vi "Execute Menu Item.vi"(7 "Device Ref in":T1 format="%.0x", 8 "error in (no error)":errorcluster, 9 "Coords":T2, 10 "ItemTag":string, 11 "CtlRef":refnum<vi>) -> (0 "error out":errorcluster)   [LabVIEW 2014, in "SLSC configuration System Explorer.lvlib"]
uses:
  SLSC configuration System Explorer.lvlib
  <vilib>/Utility/miscctls.llb/LVPoint32TypeDef.ctl
  <vilib>/NI Veristand/Custom Device API/Custom Device Item Ref.ctl
  Type Defs/Card Position.ctl
  Example/SPI Utility/Slot #.ctl
  <vilib>/NI Veristand/Custom Device Tools/Custom Device Utility Library/NI VeriStand - Search for Item by Name.vi
  <vilib>/NI Veristand/Custom Device API/Custom Device API.lvlib
  <vilib>/NI Veristand/Custom Device Tools/Custom Device Utility Library/Custom Device Utility Library.lvlib
  Shared/SLSC configuration Shared.lvlib
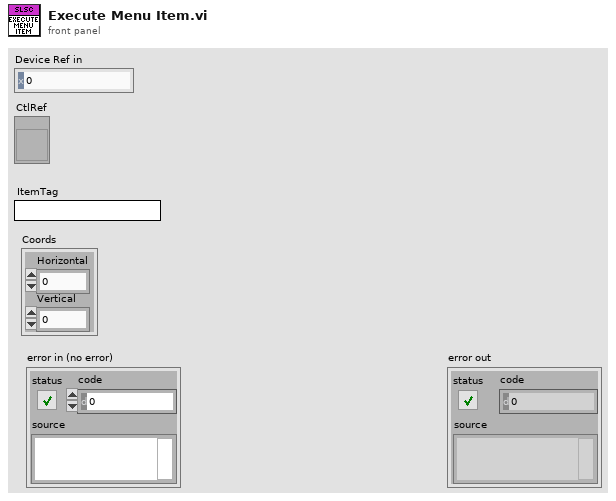
[diagram p1: front panel]
types:
  T1 = typedef "Custom Device API.lvlib/Custom Device Item Ref.ctl" = u64
  T2 = typedef "LVPoint32TypeDef.ctl" = cluster{"Horizontal":i32, "Vertical":i32}
  T3 = typedef "SLSC configuration Shared.lvlib/Card Position.ctl" = cluster{"Rack #":u8, "Slot #":T4}
  T4 = typedef "SLSC configuration Shared.lvlib/Slot #.ctl" = u8
  T5 = typedef "LVRowAndColumnTypeDef.ctl" = cluster{"Row":i32, "Column":i32}
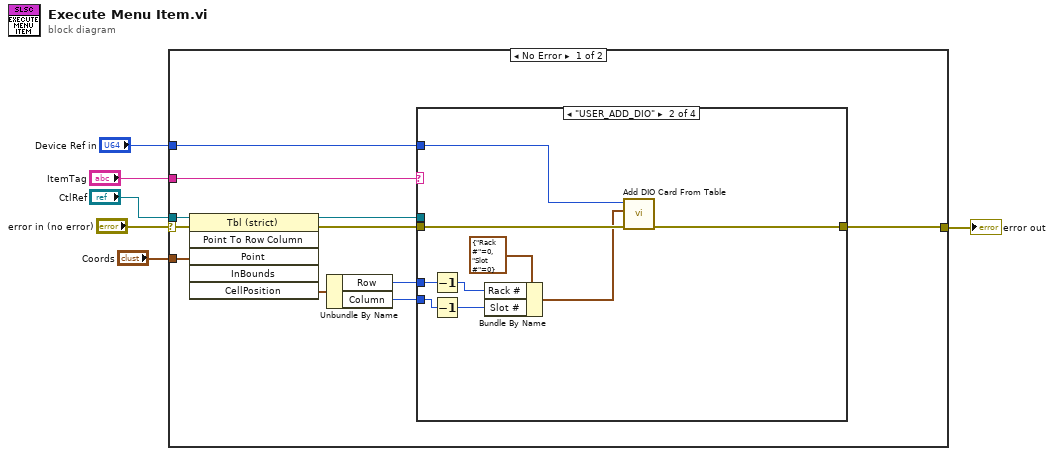
[diagram p0: block diagram]
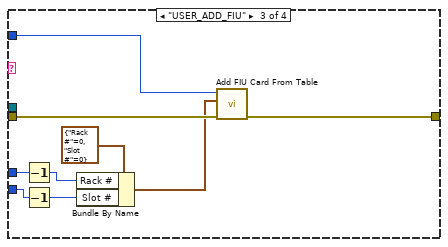
[diagram p3: hidden frame]
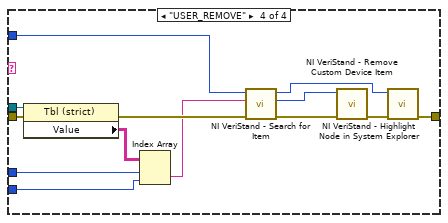
[diagram p4: hidden frame]
diagram:
  n1 = case shown="No Error" "error in (no error)" {
    selector: "error in (no error)" -> [w15 w50]
    tunnel: "ItemTag" -> [w17 _]
    tunnel: "CtlRef" -> [w16 _]
    tunnel: "Coords" -> [w14 _]
    tunnel: "Device Ref in" -> [w8 _]
    tunnel: [w7 w50] -> w1
    frame No Error {
      n2 = invoke class="Tbl (strict)" method="Point To Row Column"(reference=w16, error in=w15, "Point"=w14) -> (reference out=w13:refnum<vi>, error out=w12:errorcluster, "CellPosition"=w11:T5)  [unwired: 3 in, 3 out]
      n3 = Unbundle By Name(w11) -> ("Row"=w10:i32, "Column"=w9:i32)
      n4 = case shown="\"USER_ADD_DIO\"" w17 {
        tunnel: w13 -> [_ _ _ w49]
        tunnel: w12 -> [w18 w22 w31 w48]
        tunnel: w10 -> [_ w26 w35 w46]
        tunnel: w9 -> [_ w25 w34 w45]
        tunnel: w8 -> [_ w19 w29 w43]
        tunnel: [w18 w21 w30 w37] -> w7
        frame Default {
        }
        frame "USER_ADD_DIO" {
          n5 = Decrement(x=w26) -> (x-1=w24:i32)
          n6 = Decrement(x=w25) -> (x-1=w23:i32)
          n7 = Bundle By Name(cluster=T3 {"Rack #"=0, "Slot #"=0} ("Card Position"), "Rack #"=w24, "Slot #"=w23) -> (w20:T3)
          n8 = call "Add DIO Card From Table.vi"("error in (no error)"=w22, "Card Position"=w20, "Node Ptr"=w19) -> ("error out"=w21:errorcluster)  [unwired: 8 in]
        }
        frame "USER_ADD_FIU" {
          n9 = Decrement(x=w35) -> (x-1=w33:i32)
          n10 = Decrement(x=w34) -> (x-1=w32:i32)
          n11 = Bundle By Name(cluster=T3 {"Rack #"=0, "Slot #"=0} ("Card Position"), "Rack #"=w33, "Slot #"=w32) -> (w28:T3)
          n12 = call "Add FIU Card From Table.vi"("error in (no error)"=w31, "Card Position"=w28, "Node Ptr"=w29) -> ("error out"=w30:errorcluster)  [unwired: 8 in]
        }
        frame "USER_REMOVE" {
          n13 = property class="Tbl (strict)"(reference=w49, error in=w48) -> (error out=w44:errorcluster, "Value"=w47:string[][])  [unwired: 1 out]
          n14 = Index Array(array=w47, index (row)=w46, index (col)=w45) -> (element=w42:string)
          n15 = call-poly <vilib>:"NI VeriStand - Search for Item.vi"("error in"=w44, "Item Name"=w42, "Section Ref in"=w43) -> ("error out"=w41:errorcluster, "Item Ref"=w40:T1, "Section Ref out"=w38:T1)  [unwired: 5 in, 1 out]
          n16 = call <vilib>:"NI VeriStand - Remove Custom Device Item.vi"("error in (no error)"=w41, "Item Ref in"=w40) -> ("error out"=w39:errorcluster)  [unwired: 8 in, 1 out]
          n17 = call <vilib>:"NI VeriStand - Highlight Node in System Explorer.vi"("error in (no error)"=w39, "Item Ref in"=w38) -> ("error out"=w37:errorcluster)  [unwired: 8 in, 1 out]
        }
      }
    }
    frame Error {
    }
  }
  "error out" <- w1
